vi "Write_Hyperscope_variables_to_GFG.vi"(8 "error in (no error)":errorcluster, 10 "HyperScope Imaging Path Reso? (F)":bool, 11 "System type (Default - Standalone)":T1(ring)) -> (0 "error out":errorcluster)   [LabVIEW 2017]
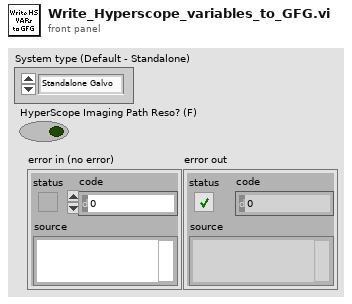
[diagram p1: front panel]
types:
  T1 = enum16{"Standalone Galvo", "Imaging Galvo", "Photostimulation Galvo"}
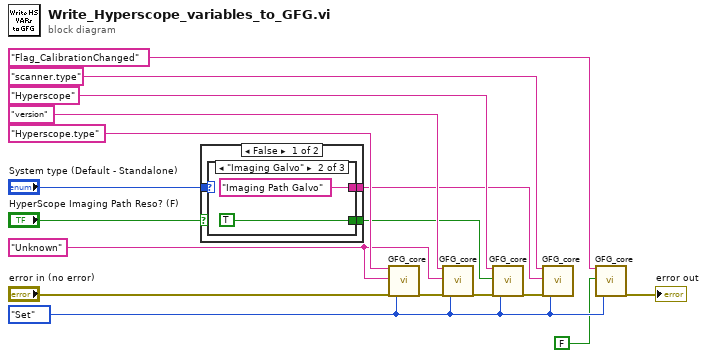
[diagram p0: block diagram]
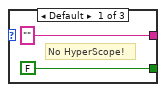
[diagram p2: hidden frame]
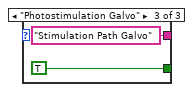
[diagram p3: hidden frame]
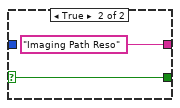
[diagram p4: hidden frame]
diagram:
  w4 = enum16{"Init", "Set", "Get", "Clear"}."Set" ("Action")
  w14 = "Unknown" ("Variable Name in")
  n1 = case shown="False" "HyperScope Imaging Path Reso? (F)" {
    selector: "HyperScope Imaging Path Reso? (F)" -> [_ w28]
    tunnel: "System type (Default - Standalone)" -> [w20 _]
    tunnel: [w19 "Imaging Path Reso" ("Variable Name in")] -> w6
    tunnel: [w18 w28] -> w7
    frame False {
      n2 = case shown="\"Imaging Galvo\"" w20 {
        tunnel: ["" ("Variable Name in") "Imaging Path Galvo" ("Variable Name in") "Stimulation Path Galvo" ("Variable Name in")] -> w19
        tunnel: [FALSE TRUE TRUE] -> w18
        frame Default {
          # "No HyperScope!"
        }
        frame "Imaging Galvo" {
        }
        frame "Photostimulation Galvo" {
        }
      }
    }
    frame True {
    }
  }
  n3 = call "GFG_core.vi"("Variable Name in"="Hyperscope.type", "Variant in"=w14, "error in (no error)"="error in (no error)", "Action"=w4) -> ("error out"=w16:errorcluster)  [unwired: 9 in, 6 out]
  n4 = call "GFG_core.vi"("Variable Name in"="version", "Variant in"=w14, "error in (no error)"=w16, "Action"=w4) -> ("error out"=w11:errorcluster)  [unwired: 9 in, 6 out]
  n5 = call "GFG_core.vi"("Variable Name in"="Hyperscope", "Variant in"=w7, "error in (no error)"=w11, "Action"=w4) -> ("error out"=w10:errorcluster)  [unwired: 9 in, 6 out]
  n6 = call "GFG_core.vi"("Variable Name in"="scanner.type", "Variant in"=w6, "error in (no error)"=w10, "Action"=w4) -> ()  [unwired: 9 in, 7 out]
  n7 = call "GFG_core.vi"("Variable Name in"="Flag_CalibrationChanged", "Variant in"=FALSE, "Action"=w4) -> ("error out"=→"error out":errorcluster)  [unwired: 10 in, 6 out]
